vi "Pharse_Param2Str (SubVI).vi"(1 "param":T1={"Time_sec"="7005.1", "HeadPow%"=0, "Temp (C)"=50}) -> (0 "param_cmd":string)   [LabVIEW 2018]
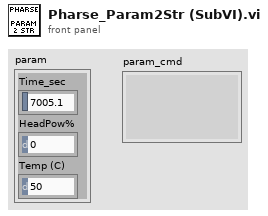
[diagram p1: front panel]
types:
  T1 = cluster{"Time_sec":string, "HeadPow%":i32, "Temp (C)":u8}
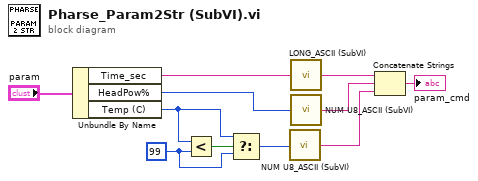
[diagram p0: block diagram]
diagram:
  w8 = u8 99 ("y")
  n1 = Unbundle By Name("param") -> ("Time_sec"=w10:string, "HeadPow%"=w1:i32, "Temp (C)"=w11:u8)
  n2 = Less?(x=w11, y=w8) -> (x < y?=w9:bool)
  n3 = Select(t=w11, s=w9, f=w8) -> (s? t:f=w2:u8)
  n4 = call "NUM U8_ASCII (SubVI).vi"("Numeric"=w2) -> ("String out"=w3:string)
  n5 = call "LONG_ASCII (SubVI).vi"("String in"=w10) -> ("String out"=w6:string)
  n6 = call "NUM U8_ASCII (SubVI).vi"("Numeric"=w1) -> ("String out"=w4:string)
  n7 = Concatenate Strings(w6, w4, w3) -> (→"param_cmd":string)
